vi "App_Connect Setting.vi"() -> ()   [LabVIEW 2015, in "Application 2.lvlib"]
uses:
  Application 2.lvlib
  Data Def/App_Config Method.ctl
  Data Def/App_Main Loop Queue Data.ctl
  Data Def/App_Subpanel Name.ctl
  Data Def/App_User Event Data.ctl
  Data Def/App_Tips Data.ctl
panel:
  in  "Connect":bool
  in  "Server IP":string caption="String"
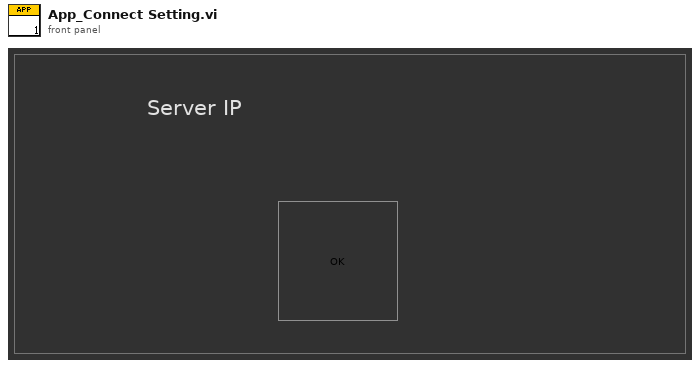
[diagram p1: front panel]
types:
  T1 = typedef "Application 2.lvlib/App_Main Loop Queue Data.ctl" = cluster{"Command":string, "Data":variant}
  T2 = typedef "Application 2.lvlib/App_Config Method.ctl" = enum16{"Get", "Put", "Load", "Save"}
  T3 = typedef "Application 2.lvlib/App_Tips Data.ctl" = cluster{"Tips":string, "BG Color":u32}
  T4 = typedef "Application 2.lvlib/App_User Event Data.ctl" = cluster{"Command":string, "Data":variant}
  T5 = typedef "Application 2.lvlib/App_Subpanel Name.ctl" = enum16{"Main", "Menu", "User Registering", "User Setting", "Monitor", "Traning Mode", "Query Data", "Connect Setting"}
  T6 = typedef "Application 2.lvlib/App_Configuration.ctl" = cluster{"Server IP":string, "User Name":string}
  T7 = typedef "Application 2.lvlib/App_Main Data.ctl" = cluster{"VI Refnum":refnum<vi>, "Subpanel":refnum<vi>, "Connection ID":refnum<k5>, "Meta data":T8[], "Main Queue":T10, "User Data":T11}
  T8 = typedef "stm_MetaElement.ctl" = cluster{"Name":T9}
  T9 = typedef "stm_MetaDataElement.ctl" = string
  T10 = typedef "Application 2.lvlib/App_Main Queue.ctl" = cluster{"Main Loop Queue":refnum<queue>}
  T11 = typedef "User Data.ctl" = cluster{"Name":string, "Email":string, "Phone Number":string, "User Picture":u32[][], "Last Login Time":timestamp}
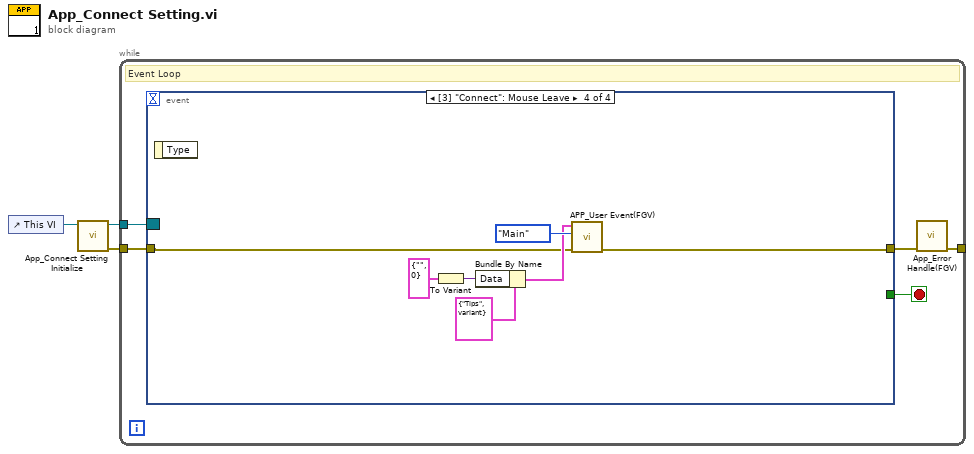
[diagram p0: block diagram]
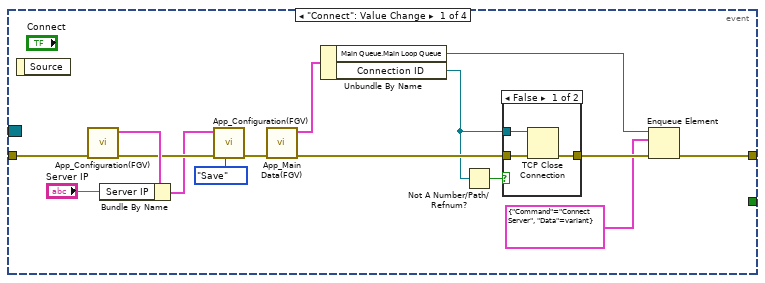
[diagram p2: hidden frame]
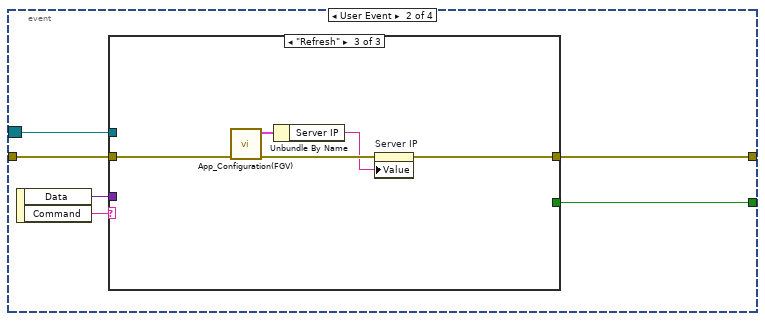
[diagram p4: hidden frame]
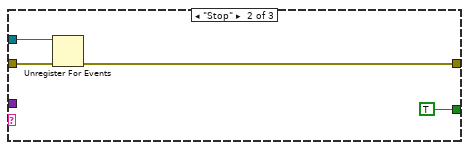
[diagram p6: hidden frame]
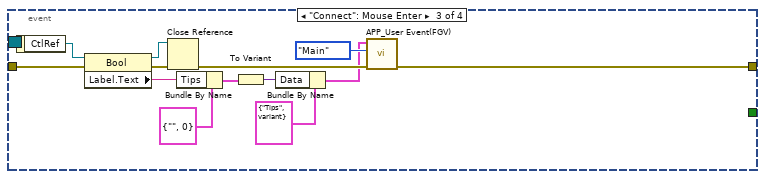
[diagram p7: hidden frame]
diagram:
  n1 = control-ref of="This VI"() -> (w3:refnum<vi>)
  n2 = call "App_Connect Setting Initialize.vi"("VI Reference"=w3) -> ("error out"=w2:errorcluster, "Event Registration Refnum"=w1:refnum<event-registration>)  [unwired: 9 in]
  n3 = while {
    tunnel: w2 -> [w8]
    tunnel: w1 -> [w7]
    tunnel: [w5] -> _
    stop <- w4 stop-if-true
    # "Event Loop"
    n4 = event shown="[3] \"Connect\": Mouse Leave" {
      selector: w7 -> [_ w29 _ _]
      dyn-events: _ -> [_ _ _ _]
      timeout: _ -> [_ _ _ _]
      tunnel: w8 -> [w23 w31 w46 w58]
      tunnel: [w11 w30 w45 w57] -> w6
      tunnel: [_ w28 _ _] -> w4
      event "Connect": Value Change {
        n5 = event-data() -> ()  [unwired: 1 in, 1 out]
        n6 = call "App_Configuration(FGV).vi"("error in"=w23) -> ("error out"=w20:errorcluster, "Configuration Out"=w22:T6)  [unwired: 9 in]
        n7 = Bundle By Name(cluster=w22, "Server IP"="Server IP") -> (w19:T6)
        n8 = call "App_Configuration(FGV).vi"("Config Method(Get)"=App_Config_Method."Save", "error in"=w20, "Configuration In"=w19) -> ("error out"=w17:errorcluster)  [unwired: 7 in, 1 out]
        n9 = call "App_Main Data(FGV).vi"("error in"=w17) -> ("error out"=w14:errorcluster, "Main Data Out"=w16:T7)  [unwired: 9 in]
        n10 = Unbundle By Name(w16) -> ("Main Queue.Main Loop Queue"=w10:refnum<queue>, "Connection ID"=w13:refnum<k5>)
        n11 = Not A Number/Path/Refnum?(number/path/refnum=w13) -> (NaN/Path/Refnum?=w15:bool)
        n12 = case shown="False" w15 {
          tunnel: w14 -> [w25 w27]
          tunnel: w13 -> [w26 _]
          tunnel: [w24 w27] -> w12
          frame False {
            n13 = TCP Close Connection(connection ID=w26, error in (no error)=w25) -> (error out=w24:errorcluster)  [unwired: 1 in, 1 out]
          }
          frame True {
          }
        }
        n14 = Enqueue Element(queue=w10, element=T1 {"Command"="Connect Server", "Data"=variant}, error in (no error)=w12) -> (error out=w11:errorcluster)  [unwired: 1 in, 2 out]
      }
      event User Event {
        n15 = event-data() -> ("Data"=w32:variant, "Command"=w33:string)  [unwired: 1 in]
        n16 = case shown="\"Refresh\"" w33 {
          tunnel: w32 -> [_ _ _]
          tunnel: w31 -> [w34 w38 w43]
          tunnel: [w34 w36 w39] -> w30
          tunnel: w29 -> [_ w37 _]
          tunnel: [_ TRUE _] -> w28
          frame Default {
          }
          frame "Stop" {
            n17 = Unregister For Events(event registration refnum=w37, error in=w38) -> (error out=w36:errorcluster)
          }
          frame "Refresh" {
            n18 = call "App_Configuration(FGV).vi"("error in"=w43) -> ("error out"=w41:errorcluster, "Configuration Out"=w42:T6)  [unwired: 9 in]
            n19 = Unbundle By Name(w42) -> ("Server IP"=w40:string)
            n20 = property on="Server IP" class="Str"(error in=w41, "Value"=w40) -> (error out=w39:errorcluster)  [unwired: 1 in, 1 out]
          }
        }
      }
      event "Connect": Mouse Enter {
        n21 = event-data() -> ("CtlRef"=w44:refnum<vi>)  [unwired: 1 in]
        n22 = property class="Bool"(reference=w44, error in=w46) -> (reference out=w55:refnum<vi>, error out=w56:errorcluster, "Label.Text"=w48:string)
        n23 = Close Reference(reference=w55, error in (no error)=w56) -> (error out=w53:errorcluster)
        n24 = Bundle By Name(cluster=T3 {"Tips"="", "BG Color"=0} ("Tips Data"), "Tips"=w48) -> (w47:T3)
        n25 = To Variant(anything=w47) -> (Variant=w51:variant)
        n26 = Bundle By Name(cluster=T4 {"Command"="Tips", "Data"=variant} ("User Event Data"), "Data"=w51) -> (w50:T4)
        n27 = call "APP_User Event(FGV).vi"("error in"=w53, "Subpanel Name"=App_Subpanel_Name."Main", "User Event Data"=w50) -> ("error out"=w45:errorcluster)  [unwired: 7 in, 1 out]
      }
      event "Connect": Mouse Leave {
        n28 = event-data() -> ()  [unwired: 1 in, 1 out]
        n29 = To Variant(anything=T3 {"Tips"="", "BG Color"=0} ("Tips Data")) -> (Variant=w61:variant)
        n30 = Bundle By Name(cluster=T4 {"Command"="Tips", "Data"=variant} ("User Event Data"), "Data"=w61) -> (w60:T4)
        n31 = call "APP_User Event(FGV).vi"("error in"=w58, "Subpanel Name"=App_Subpanel_Name."Main", "User Event Data"=w60) -> ("error out"=w57:errorcluster)  [unwired: 7 in, 1 out]
      }
    }
    n32 = call "App_Error Handle(FGV).vi"("error in"=w6) -> ("error out"=w5:errorcluster)  [unwired: 9 in, 1 out]
  }
